vi "Set Stopped.vi"(8 "error in (no error)":errorcluster caption="entrée d'erreur (pas d'erreur)", 10 "Stopped":bool, 11 "Actor Test (Default) en entrée":refnum<class "Actor Test (Default).lvclass">) -> (0 "error out":errorcluster caption="sortie d'erreur", 3 "Actor Test (Default) en sortie":refnum<class "Actor Test (Default).lvclass">)   [LabVIEW 2020, in "Library Core.lvlib" / "Actor Test (Default).lvclass"]
uses:
  Actor Test (Default).lvclass
  Actor Test (Default).lvclass/Actor Test (Default).ctl
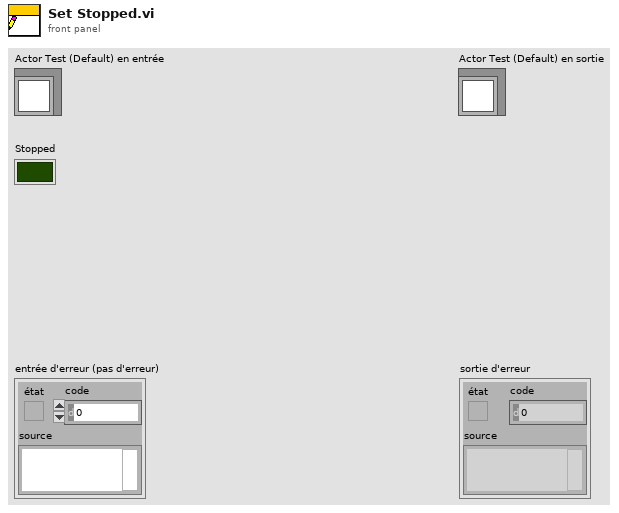
[diagram p1: front panel]
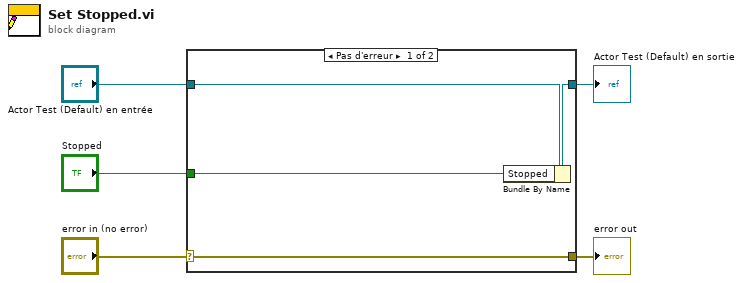
[diagram p0: block diagram]
diagram:
  n1 = case shown="Pas d'erreur" "error in (no error)" {
    selector: "error in (no error)" -> [w9 w10]
    tunnel: [w9 w10] -> w4
    tunnel: [w7 w11] -> w2
    tunnel: "Actor Test (Default) en entrée" -> [w8 w11]
    tunnel: "Stopped" -> [w6 _]
    frame No Error {
      n2 = Bundle By Name(cluster=w8, "Stopped"=w6) -> (w7:refnum<class "Actor Test (Default).lvclass">)
    }
    frame Error {
    }
  }
  "error out" <- w4
  "Actor Test (Default) en sortie" <- w2
